vi "Init Device.vi"(8 "error in (no error)":errorcluster, 11 "Device in":refnum<class "PIC-Device.lvclass">) -> (0 "error out":errorcluster, 3 "Device out":refnum<class "PIC-Device.lvclass">)   [LabVIEW 2020, in "PIC-Device.lvclass"]
doc: "Init the device com port.\nThis should be called by the child class and the child class is responsible for setting the device as its default state."
uses:
  PIC-Device.lvclass
  C:/Sandbox/Git_Sandbox/WiSpry Test Framework source code (LV20)/WiSpry Test Framework/Devices/Device.lvclass
  <vilib>/Instr/_visa.llb/Select Event Type.ctl
  PIC-Device.lvclass/PIC-Device.ctl
  <vilib>/Instr/_visa.llb/VISA Configure Serial Port (Instr).vi
  Device.lvclass
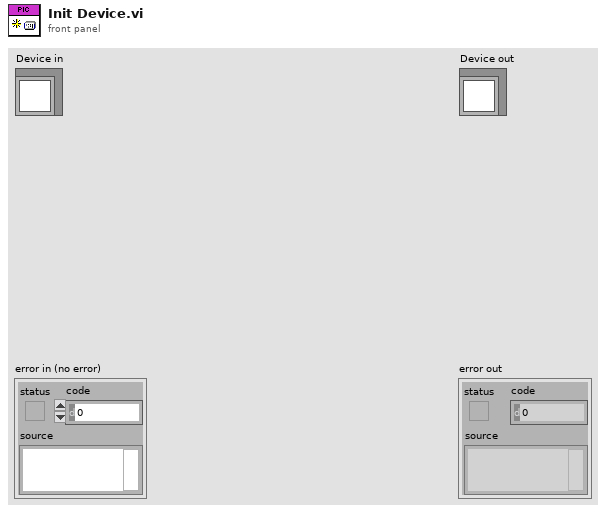
[diagram p1: front panel]
types:
  T1 = typedef "Select Event Type.ctl" = u32
  T2 = enum16{"RFFE 2-wire", "WiSPI 3-wire spi_sel", "WiSPI 4-wire spi_sel", "ifxSPI 3-wire spi_sel", "WiSPI 3-wire dev add spi_sel"}
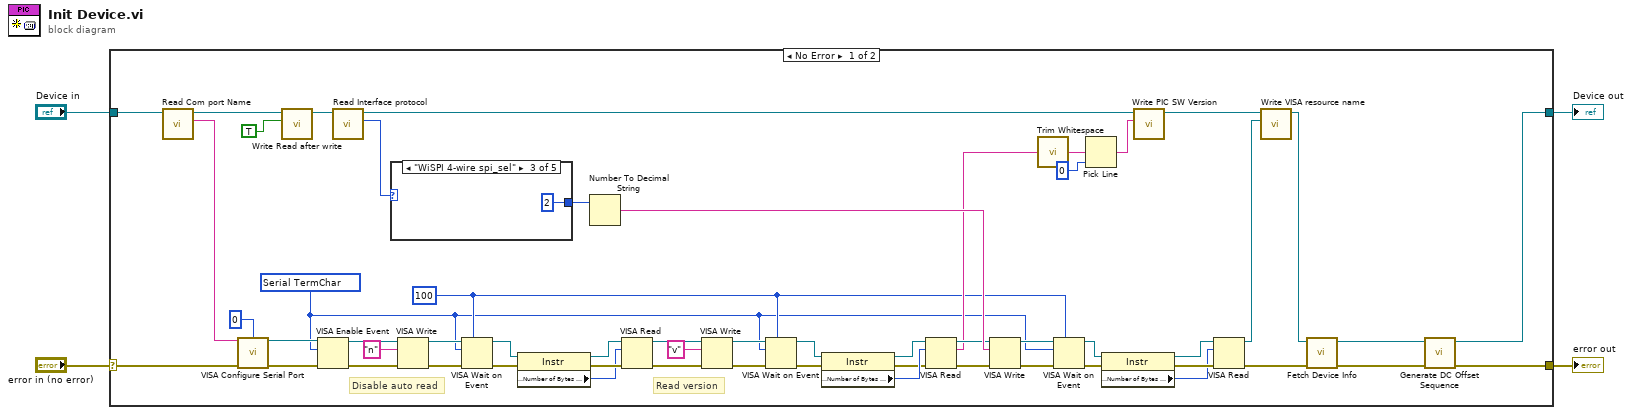
[diagram p0: block diagram]
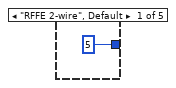
[diagram p2: hidden frame]
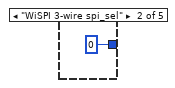
[diagram p3: hidden frame]
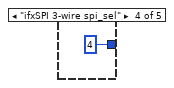
[diagram p4: hidden frame]
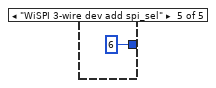
[diagram p5: hidden frame]
diagram:
  n1 = case shown="No Error" "error in (no error)" {
    selector: "error in (no error)" -> [w59 w67]
    tunnel: [w13 w67] -> w3
    tunnel: [w8 w66] -> w1
    tunnel: "Device in" -> [w60 w66]
    frame No Error {
      w18 = u32 100 ("timeout (0)")
      w17 = T1 1073684516 items=["Service Request"=1073684491, "Trigger"=3221168138, "Clear"=1073684493, "VXI Signal"=1073684512, "VXI/VME Interrupt"=3221168161, "VXI/VME Sysfail"=1073684509, "VXI/VME Sysreset"=1073684510, "GPIB CIC"=1073684498, "GPIB Talk"=1073684499, "GPIB Listen"=1073684500, "PXI Interrupt"=1073684514, "Serial Break"=1073684515, "Serial TermChar"=1073684516, "Serial CTS"=1073684521, "Serial DSR"=1073684522, "Serial DCD"=1073684524, "Serial RI"=1073684526, "Serial Character"=1073684533, "USB Interrupt"=1073684535, "All Enabled"=1073709055] ("Event Type")
      # "Read version"
      # "Disable auto read"
      n2 = call "Read Com port Name.vi"("Device in"=w60) -> ("Com port Name"=w58:string, "Device out"=w7:refnum<class "PIC-Device.lvclass">)  [unwired: 9 in]
      n3 = call-poly "VISA Configure Serial Port"("VISA resource name"=w58, "termination char\n(0xA = '\\n' = LF)"=u8 0 ("termination char\n(0xA = '\\n' = LF)"), "error in (no error)"=w59) -> ("VISA resource name out"=w55:refnum<visa-resource-name>, "error out"=w56:errorcluster)  [unwired: 11 in]
      n4 = call-dynamic "Write Read after write.vi"("Read after write"=TRUE, "Device in"=w7) -> ("Device out"=w6:refnum<class "PIC-Device.lvclass">)  [unwired: 9 in]
      n5 = VISA Enable Event(8:w56, 10:w17, 11:w55) -> (0:w54:errorcluster, 3:w53:refnum<visa-resource-name>)  [unwired: 1 in]
      n6 = call-dynamic "Read Interface protocol.vi"("Device in"=w6) -> ("Interface protocol"=w36:T2, "Device out"=w20:refnum<class "PIC-Device.lvclass">)  [unwired: 9 in]
      n7 = case shown="\"WiSPI 4-wire spi_sel\"" w36 {
        tunnel: [5 0 2 4 6] -> w35
        frame "RFFE 2-wire", Default {
        }
        frame "WiSPI 3-wire spi_sel" {
        }
        frame "WiSPI 4-wire spi_sel" {
        }
        frame "ifxSPI 3-wire spi_sel" {
        }
        frame "WiSPI 3-wire dev add spi_sel" {
        }
      }
      n8 = VISA Write(VISA resource name=w53, write buffer="n", error in (no error)=w54) -> (VISA resource name out=w50:refnum<visa-resource-name>, error out=w51:errorcluster)  [unwired: 1 out]
      n9 = VISA Wait on Event(7:w18, 8:w51, 10:w17, 11:w50) -> (0:w48:errorcluster, 3:w49:refnum<visa-resource-name>)  [unwired: 1 in, 2 out]
      n10 = property class="Instr"(reference=w49, error in=w48) -> (reference out=w45:refnum<visa-resource-name>, error out=w47:errorcluster, "Serial Settings:Number of Bytes at Serial Port"=w46:u32)
      n11 = Number To Decimal String(number=w35) -> (decimal integer string=w34:string)  [unwired: 1 in]
      n12 = VISA Read(VISA resource name=w45, byte count=w46, error in (no error)=w47) -> (VISA resource name out=w25:refnum<visa-resource-name>, error out=w24:errorcluster)  [unwired: 2 out]
      n13 = VISA Write(VISA resource name=w25, write buffer="v", error in (no error)=w24) -> (VISA resource name out=w28:refnum<visa-resource-name>, error out=w27:errorcluster)  [unwired: 1 out]
      n14 = VISA Wait on Event(7:w18, 8:w27, 10:w17, 11:w28) -> (0:w30:errorcluster, 3:w29:refnum<visa-resource-name>)  [unwired: 1 in, 2 out]
      n15 = property class="Instr"(reference=w29, error in=w30) -> (reference out=w33:refnum<visa-resource-name>, error out=w31:errorcluster, "Serial Settings:Number of Bytes at Serial Port"=w32:u32)
      n16 = VISA Read(VISA resource name=w33, byte count=w32, error in (no error)=w31) -> (VISA resource name out=w22:refnum<visa-resource-name>, read buffer=w19:string, error out=w23:errorcluster)  [unwired: 1 out]
      n17 = VISA Write(VISA resource name=w22, write buffer=w34, error in (no error)=w23) -> (VISA resource name out=w43:refnum<visa-resource-name>, error out=w44:errorcluster)  [unwired: 1 out]
      n18 = call <vilib>:"Trim Whitespace.vi"("string"=w19) -> ("trimmed string"=w16:string)  [unwired: 1 in]
      n19 = VISA Wait on Event(7:w18, 8:w44, 10:w17, 11:w43) -> (0:w41:errorcluster, 3:w42:refnum<visa-resource-name>)  [unwired: 1 in, 2 out]
      n20 = Pick Line(multi-line string=w16, line index=0) -> (output string=w14:string)  [unwired: 1 in]
      n21 = property class="Instr"(reference=w42, error in=w41) -> (reference out=w38:refnum<visa-resource-name>, error out=w40:errorcluster, "Serial Settings:Number of Bytes at Serial Port"=w39:u32)
      n22 = call "Write PIC SW Version.vi"("PIC SW Version"=w14, "Device in"=w20) -> ("Device out"=w21:refnum<class "PIC-Device.lvclass">)  [unwired: 9 in]
      n23 = VISA Read(VISA resource name=w38, byte count=w39, error in (no error)=w40) -> (VISA resource name out=w37:refnum<visa-resource-name>, error out=w12:errorcluster)  [unwired: 2 out]
      n24 = call-dynamic "Write VISA resource name.vi"("VISA resource name"=w37, "Device in"=w21) -> ("Device out"=w9:refnum<class "PIC-Device.lvclass">)  [unwired: 9 in]
      n25 = call-dynamic "Fetch Device Info.vi"("error in (no error)"=w12, "PIC-Device in"=w9) -> ("error out"=w11:errorcluster, "PIC-Device out"=w10:refnum<class "PIC-Device.lvclass">)  [unwired: 7 in, 1 out]
      n26 = call "Generate DC Offset Sequence.vi"("error in (no error)"=w11, "Device in"=w10) -> ("error out"=w13:errorcluster, "Device out"=w8:refnum<class "PIC-Device.lvclass">)  [unwired: 8 in]
    }
    frame Error {
    }
  }
  "error out" <- w3
  "Device out" <- w1
